vi "Write configuration.vi"(8 "error in":errorcluster, 10 "configuration":refnum<class "NISE_CEF_serializable configuration.lvclass">, 11 "Getting Started IO editor node in":refnum<class "io editor node.lvclass">) -> (0 "error out":errorcluster, 3 "Getting Started IO editor node out":refnum<class "io editor node.lvclass">)   [LabVIEW 2014, in "io editor node.lvclass"]
uses:
  io editor node.lvclass
  configuration/io configuration.lvclass
  <vilib>/NI/Configuration Framework/serializable configuration/NISE_CEF_serializable configuration.lvclass
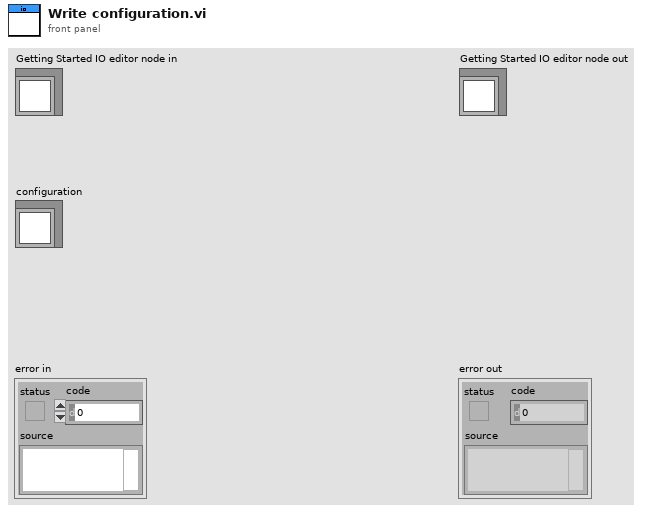
[diagram p1: front panel]
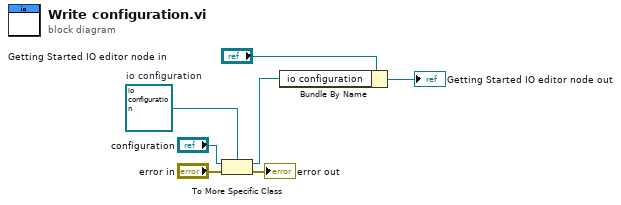
[diagram p0: block diagram]
diagram:
  w1 = refnum<class "io configuration.lvclass"> refnum  # io configuration
  n1 = To More Specific Class(target class=w1, reference="configuration", error in="error in") -> (specific class reference=w2:refnum<class "io configuration.lvclass">, error out=→"error out":errorcluster)
  n2 = Bundle By Name(cluster="Getting Started IO editor node in", "io configuration"=w2) -> (→"Getting Started IO editor node out":refnum<class "io editor node.lvclass">)
